vi "CEchoSCU.vi"() -> ()   [LabVIEW 2013]
panel:
  out "String":string="C:\\Users\\Simon\\Dropbox\\Medimatic\\Project Ver. LV2011\\DICOM\\dcmtk\\bin\\echoscu.exe -v -aet SCU -aec ANY-SCP www.dicomserver.co.uk 11112"
  out "return code":i32
  in  "port":string="11112"
  in  "server(ip)":string="www.dicomserver.co.uk "
  in  "aec":string="ANY-SCP"
  in  "aet":string="SCU"
  in  "standard input":string
  in  "executable path":string="C:\\Users\\Simon\\Dropbox\\Medimatic\\Project Ver. LV2011\\DICOM\\dcmtk\\bin\\echoscu.exe"
  in  "error in (no error)":errorcluster
  out "error out":errorcluster
  out "standard error":string
  out "standard output":string
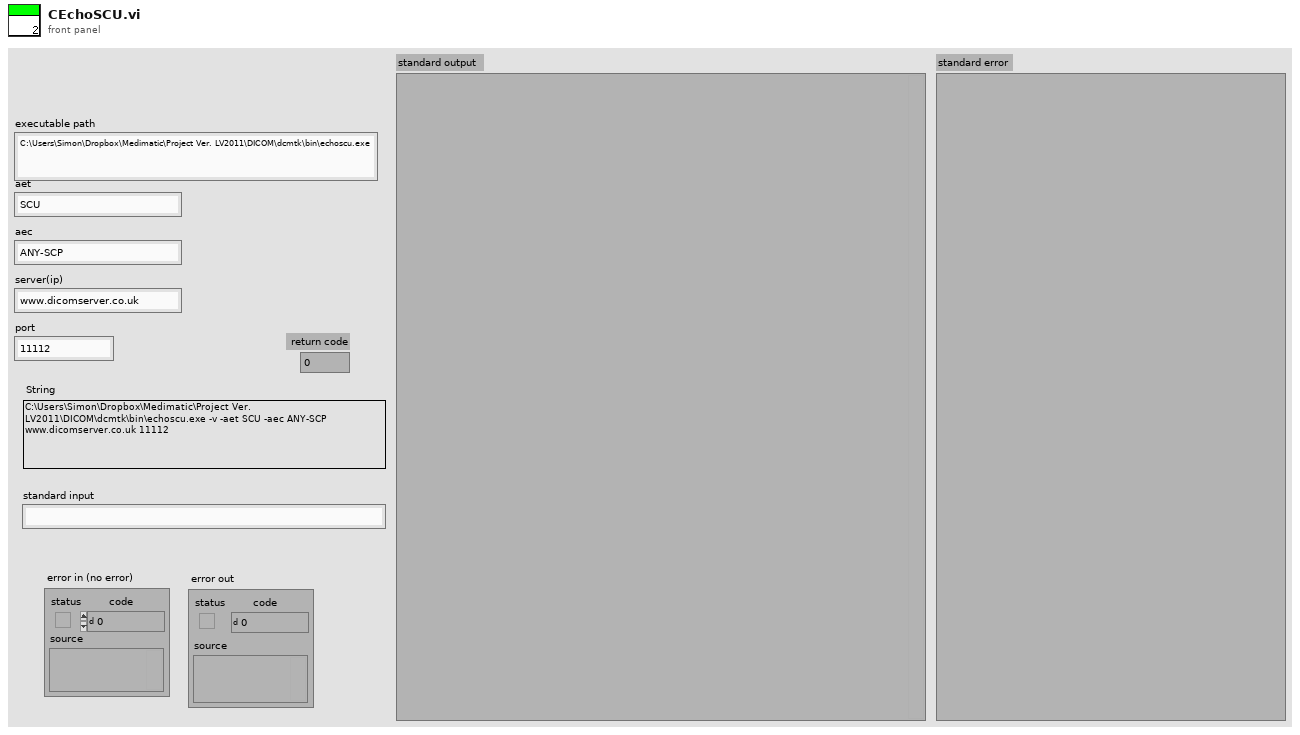
[diagram p1: front panel]
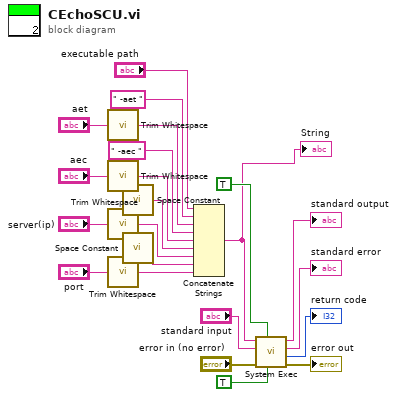
[diagram p0: block diagram]
diagram:
  n1 = call <vilib>:"Trim Whitespace.vi"("string"="aet") -> ("trimmed string"=w11:string)  [unwired: 1 in]
  n2 = call <vilib>:"Trim Whitespace.vi"("string"="aec") -> ("trimmed string"=w9:string)  [unwired: 1 in]
  n3 = call <vilib>:"Trim Whitespace.vi"("string"="server(ip)") -> ("trimmed string"=w3:string)  [unwired: 1 in]
  n4 = call <vilib>:"Trim Whitespace.vi"("string"="port") -> ("trimmed string"=w5:string)  [unwired: 1 in]
  n5 = call <vilib>:"Space Constant.vi"() -> ("String"=w8:string)
  n6 = call <vilib>:"Space Constant.vi"() -> ("String"=w7:string)
  n7 = Concatenate Strings("executable path", " -aet " ("string"), w11, " -aec " ("string"), w9, w8, w3, w7, w5) -> (w1:string)
  "String" <- w1
  n8 = call <vilib>:"System Exec.vi"("run minimized? (F)"=TRUE, "wait until completion? (T)"=TRUE, "error in (no error)"="error in (no error)", "standard input"="standard input", "command line"=w1) -> ("error out"=→"error out":errorcluster, "return code"=→"return code":i32, "standard error"=→"standard error":string, "standard output"=→"standard output":string)  [unwired: 3 in]
